vi "gotoB.vi"(8 "error in (no error)":errorcluster, 9 "Heater":bool, 10 "Sweeprate (T/min)":dbl, 11 "Target Field (T)":dbl) -> (0 "error out":errorcluster)   [LabVIEW 2009]
uses:
  Instance           1 13Saved   gotoB .vi
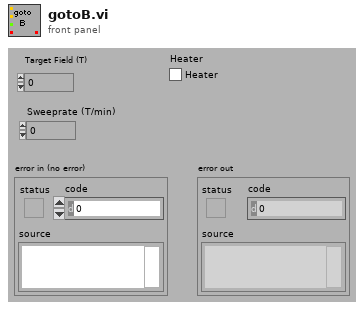
[diagram p1: front panel]
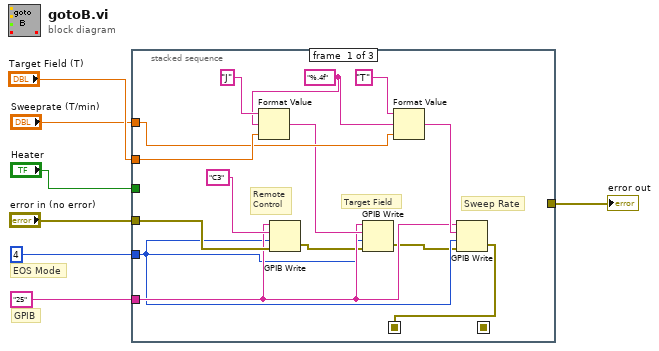
[diagram p0: block diagram]
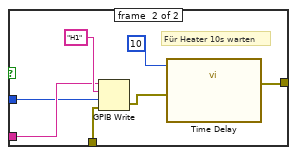
[diagram p3: hidden frame]
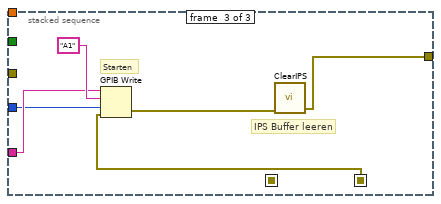
[diagram p4: hidden frame]
diagram:
  # "GPIB"
  # "EOS Mode"
  n1 = stacked-sequence {
    seq-local: [w8 _ _] -> [_ w23 _]
    seq-local: [_ w22 _] -> [_ _ w37]
    tunnel: "25" -> [w12 w25 w39]
    tunnel: 4 -> [w11 w24 w38]
    tunnel: "error in (no error)" -> [w20 _ _]
    tunnel: "Target Field (T)" -> [w16 _ _]
    tunnel: "Sweeprate (T/min)" -> [w15 _ _]
    tunnel: "Heater" -> [_ w26 _]
    tunnel: [_ _ w35] -> w1
    frame #0 {
      w17 = "%.4f"
      # "Sweep Rate"
      # "Target Field"
      # "Remote\nControl"
      n2 = Format Value(string ("")="J", format string=w17, value (0)=w16) -> (output string=w14:string)
      n3 = GPIB Write(0:w12, 1:"C3", 2:w11, 3:w20) -> (6:w10:errorcluster)  [unwired: 1 in, 1 out]
      n4 = GPIB Write(0:w12, 1:w14, 2:w11, 3:w10) -> (6:w9:errorcluster)  [unwired: 1 in, 1 out]
      n5 = Format Value(string ("")="T", format string=w17, value (0)=w15) -> (output string=w13:string)
      n6 = GPIB Write(0:w12, 1:w13, 2:w11, 3:w9) -> (6:w8:errorcluster)  [unwired: 1 in, 1 out]
    }
    frame #1 {
      n7 = case shown="True" w26 {
        tunnel: w25 -> [_ w33]
        tunnel: w24 -> [_ w32]
        tunnel: w23 -> [w27 w31]
        tunnel: [w27 w29] -> w22
        frame #0 {
        }
        frame #1 {
          # "Für Heater 10s warten"
          n8 = GPIB Write(0:w33, 1:"H1", 2:w32, 3:w31) -> (6:w30:errorcluster)  [unwired: 1 in, 1 out]
          n9 = call "Time Delay"("error in (no error)"=w30, "Delay Time (s)"=10) -> ("error out"=w29:errorcluster)  [unwired: 9 in]
        }
      }
    }
    frame #2 {
      # "IPS Buffer leeren"
      # "Starten"
      n10 = GPIB Write(0:w39, 1:"A1", 2:w38, 3:w37) -> (6:w36:errorcluster)  [unwired: 1 in, 1 out]
      n11 = call "ClearIPS.vi"("error in (no error)"=w36) -> ("error out"=w35:errorcluster)  [unwired: 4 in]
    }
  }
  "error out" <- w1
